vi "Bundle.vi"(8 "error in (no error)":errorcluster, 9 "Data Values":variant[](array[variant]), 10 "Control Indices":i32[](array[numeric]), 11 "Set Controls in":refnum<class "Set Controls.lvclass">) -> (0 "error out":errorcluster, 3 "Set Controls out":refnum<class "Set Controls.lvclass">)   [LabVIEW 2020, in "Msg.lvlib" / "Set Controls.lvclass"]
doc: "Write Control Indices and Data Values to the class private data."
uses:
  Set Controls.lvclass
  Set Controls.lvclass/Set Controls.ctl
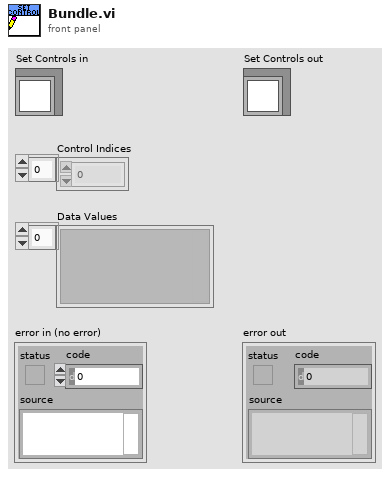
[diagram p1: front panel]
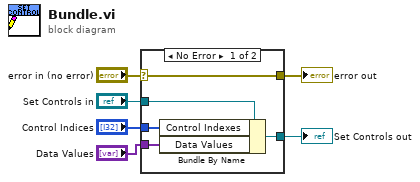
[diagram p0: block diagram]
diagram:
  n1 = case shown="No Error" "error in (no error)" {
    selector: "error in (no error)" -> [w11 w12]
    tunnel: [w11 w12] -> w5
    tunnel: [w9 w13] -> w3
    tunnel: "Set Controls in" -> [w10 w13]
    tunnel: "Control Indices" -> [w8 _]
    tunnel: "Data Values" -> [w7 _]
    frame No Error {
      n2 = Bundle By Name(cluster=w10, "Control Indexes"=w8, "Data Values"=w7) -> (w9:refnum<class "Set Controls.lvclass">)
    }
    frame Error {
    }
  }
  "error out" <- w5
  "Set Controls out" <- w3
